vi "AutoDrive.vi"(6 "Distance (Inches)":dbl, 7 "GyroDevRef":T6={"DevStatus"={"status"=FALSE, "code"=0, "source"=""}, "Analog Channel"=enum."AI 0", "Gain (VoltsPerDegree/Second)"=0.0, "Gyro Type"=enum."Analog", "Handle"=0, "SPI Bus"=enum."Invalid", "Device Found"=FALSE, "Sample Rate"=1.0, "Calibrate On Open"=FALSE, "Offset"=0.0} {"Sample Rate" min=0.25 max=100.0 step=0.25}, 8 "error in":errorcluster, 9 "LeftDevRef":T1={"DeviceStatus"={"status"=FALSE, "code"=0, "source"=""}, "Type"=enum."PWM", "PWM"={"PWM Channel"=enum."PWM 1", "DeadBand"={"Name"="", "maxPositivePwm"=0, "minPositivePwm"=0, "centerPwm"=0, "maxNegativePwm"=0, "minNegativePwm"=0, "angularRange"=0}}, "CAN"={"Device Number"=0, "SetOutput VI Ref"=variant(enum8{"Percent VBus", "Current", "Speed", "Position", "Voltage"} enum."Percent VBus"), "GetOutput VI Ref"=variant(refnum<k1> refnum), "Enable VI Ref"=variant(dbl 12.0), "Disable VI Ref"=variant(enum8{"Percent VBus", "Speed", "Position", "Slave", "Unchanged / Invalid", "Voltage Compensation", "Current", "Motion Profile"} enum."Percent VBus"), "Data"=variant}, "Invert"=FALSE, "DIO PWM"={"PWM \"Enable\" Channel"=enum."Invalid", "DIOChannel"=enum."Invalid", "PWM Rate"=0.0}}, 10 "RightDevRef":T1={"DeviceStatus"={"status"=FALSE, "code"=0, "source"=""}, "Type"=enum."PWM", "PWM"={"PWM Channel"=enum."PWM 1", "DeadBand"={"Name"="", "maxPositivePwm"=0, "minPositivePwm"=0, "centerPwm"=0, "maxNegativePwm"=0, "minNegativePwm"=0, "angularRange"=0}}, "CAN"={"Device Number"=0, "SetOutput VI Ref"=variant(enum8{"Percent VBus", "Current", "Speed", "Position", "Voltage"} enum."Percent VBus"), "GetOutput VI Ref"=variant(refnum<k1> refnum), "Enable VI Ref"=variant(dbl 12.0), "Disable VI Ref"=variant(enum8{"Percent VBus", "Speed", "Position", "Slave", "Unchanged / Invalid", "Voltage Compensation", "Current", "Motion Profile"} enum."Percent VBus"), "Data"=variant}, "Invert"=FALSE, "DIO PWM"={"PWM \"Enable\" Channel"=enum."Invalid", "DIOChannel"=enum."Invalid", "PWM Rate"=0.0}}, 11 "DriveDevRef":T9={"DevStatus"={"status"=FALSE, "code"=0, "source"=""}, "Motors[]"=[], "Square Inputs"=FALSE, "Max Output"=1.0}) -> (0 "error out":errorcluster)   [LabVIEW 2017]
uses:
  <vilib>/Rock Robotics/WPI/RobotDrive/WPI_RobotDriveDevRef.ctl
  <vilib>/Rock Robotics/WPI/MotorControl/WPI_MotorControlDeviceRef.ctl
  <vilib>/Rock Robotics/WPI/MotorControl/WPI_MotorControlType.ctl
  <vilib>/Rock Robotics/SystemInterfaces/DIO/FPGA_DIOPWMChannel.ctl
  <vilib>/Rock Robotics/WPI/PWM/WPI_PWMDeadband.ctl
  <vilib>/Rock Robotics/SystemInterfaces/DIO/FPGA_DIOChannel.ctl
  <vilib>/Rock Robotics/WPI/Gyro/WPI_GyroDevRef.ctl
  <vilib>/Rock Robotics/SystemInterfaces/AI/FPGA_AIChannel.ctl
  <vilib>/Rock Robotics/SystemInterfaces/spilib/spi_bus.ctl
  <vilib>/Rock Robotics/WPI/ThirdParty/Phoenix-LabVIEW/Motor Controller/Get/CTRE_Phoenix_MotorController_GetQuadratureData.vi
  <vilib>/Rock Robotics/WPI/RobotDrive/WPI_RobotDriveArcadeDrive_Standard(NoSaturation).vi
panel:
  # "Analog"
  # "XRS"
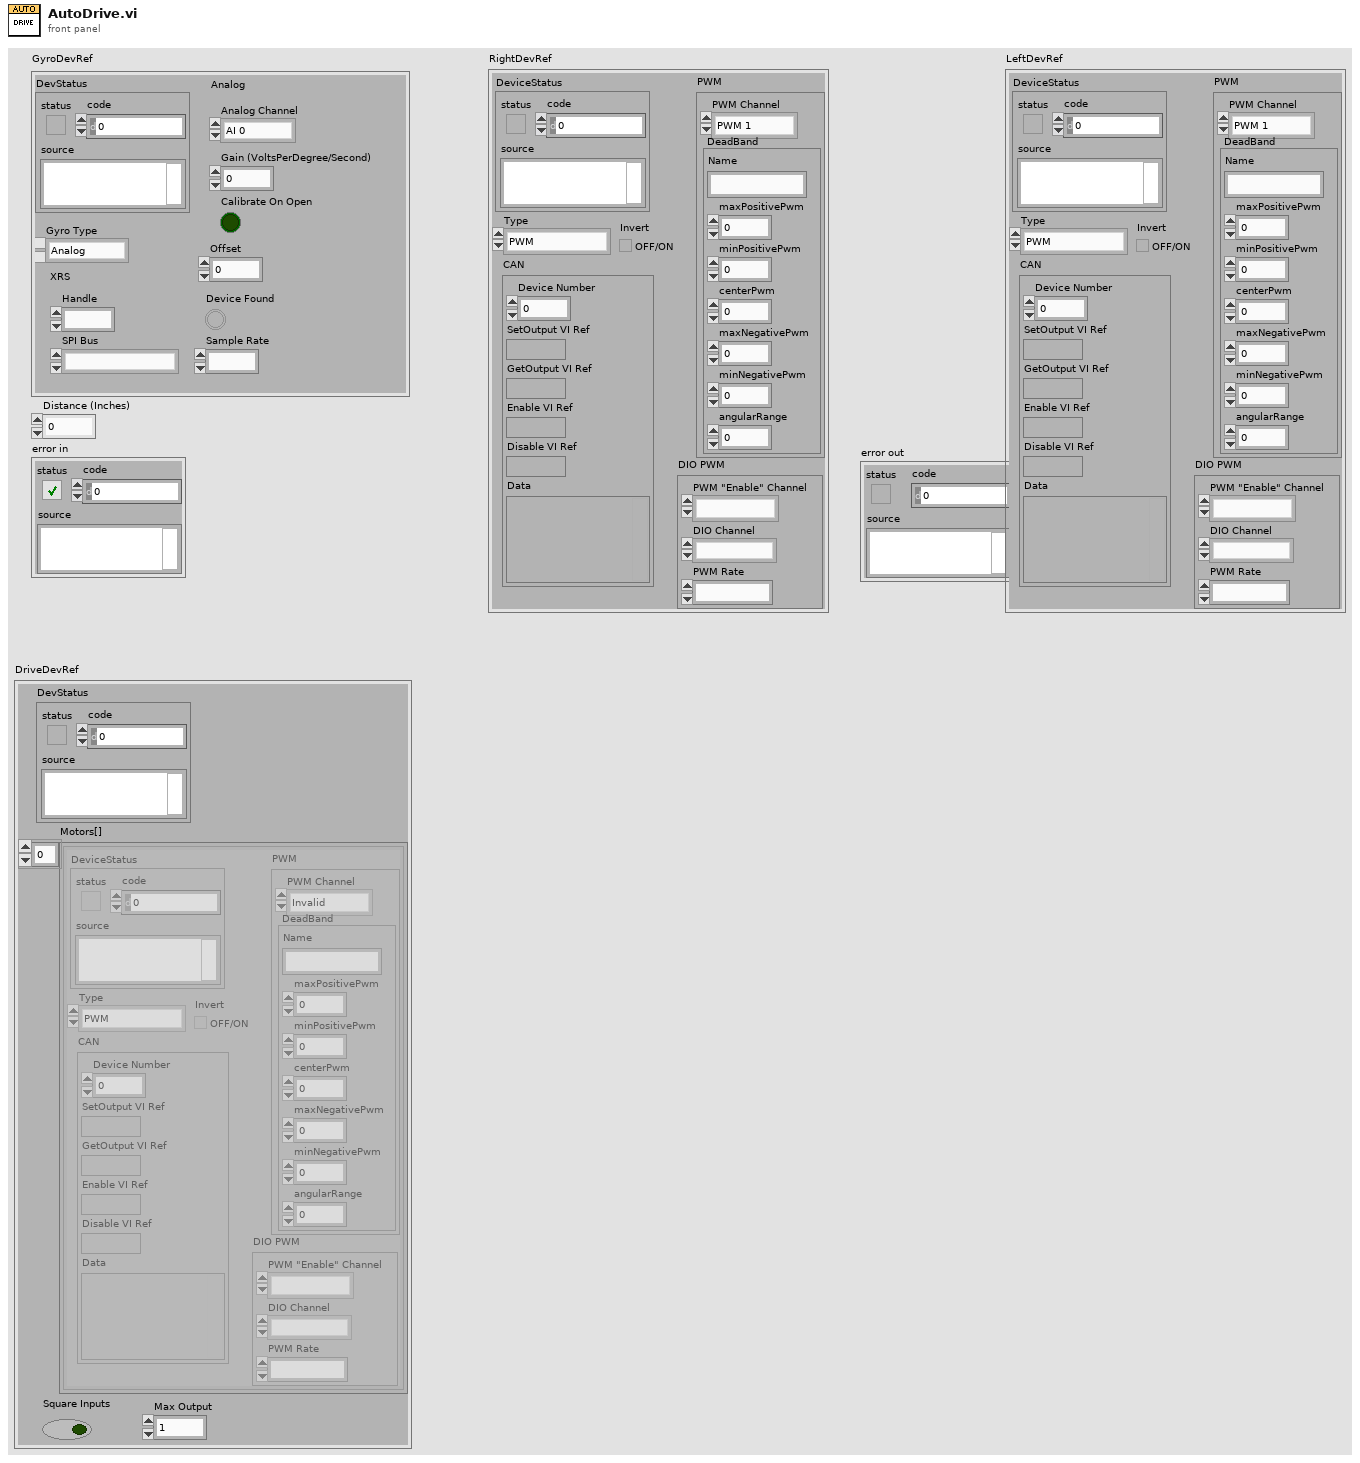
[diagram p1: front panel]
types:
  T1 = typedef "WPI_MotorControlDeviceRef.ctl" = cluster{"DeviceStatus":errorcluster, "Type":T2, "PWM":cluster{"PWM Channel":T3, "DeadBand":T4}, "CAN":cluster{"Device Number":u8, "SetOutput VI Ref":variant, "GetOutput VI Ref":variant, "Enable VI Ref":variant, "Disable VI Ref":variant, "Data":variant}, "Invert":bool, "DIO PWM":cluster{"PWM \"Enable\" Channel":T3, "DIOChannel":T5, "PWM Rate":dbl}}
  T2 = typedef "WPI_MotorControlType.ctl" = enum16{"PWM", "CAN", "DIO PWM"}
  T3 = typedef "FPGA_DIOPWMChannel.ctl" = enum8{"PWM 0", "PWM 1", "PWM 2", "PWM 3", "PWM 4", "PWM 5", "PWM 6", "PWM 7", "PWM 8", "PWM 9", "PWM MXP 0", "PWM MXP 1", "PWM MXP 2", "PWM MXP 3", "PWM MXP 4", "PWM MXP 5", "PWM MXP 6", "PWM MXP 7", "PWM MXP 8", "PWM MXP 9", "Invalid"}
  T4 = typedef "WPI_PWMDeadband.ctl" = cluster{"Name":string, "maxPositivePwm":i32, "minPositivePwm":i32, "centerPwm":i32, "maxNegativePwm":i32, "minNegativePwm":i32, "angularRange":u16}
  T5 = typedef "FPGA_DIOChannel.ctl" = enum8{"DIO 0", "DIO 1", "DIO 2", "DIO 3", "DIO 4", "DIO 5", "DIO 6", "DIO 7", "DIO 8", "DIO 9", "DIO MXP 0", "DIO MXP 1", "DIO MXP 2", "DIO MXP 3", "DIO MXP 4", "DIO MXP 5", "DIO MXP 6", "DIO MXP 7", "DIO MXP 8", "DIO MXP 9", "DIO MXP 10", "DIO MXP 11", "DIO MXP 12", "DIO MXP 13", "DIO MXP 14", "DIO MXP 15", "SPI Port CS1", "SPI Port CS2", "SPI Port CS3", "SPI Port MISO", "SPI Port MOSI", "Invalid"}
  T6 = typedef "WPI_GyroDevRef.ctl" = cluster{"DevStatus":errorcluster, "Analog Channel":T7, "Gain (VoltsPerDegree/Second)":dbl, "Gyro Type":enum16{"Analog", "XRS450"}, "Handle":i32, "SPI Bus":T8, "Device Found":bool, "Sample Rate":dbl, "Calibrate On Open":bool, "Offset":dbl}
  T7 = typedef "FPGA_AIChannel.ctl" = enum8{"AI 0", "AI 1", "AI 2", "AI 3", "AI MXP 0", "AI MXP 1", "AI MXP 2", "AI MXP 3", "Invalid"}
  T8 = typedef "spi_bus.ctl" = enum16{"SPI On-Board, CS0", "SPI On-Board, CS1", "SPI On-Board, CS2", "SPI On-Board, CS3", "SPI MXP", "Invalid"}
  T9 = typedef "WPI_RobotDriveDevRef.ctl" = cluster{"DevStatus":errorcluster, "Motors[]":T1[], "Square Inputs":bool, "Max Output":dbl}
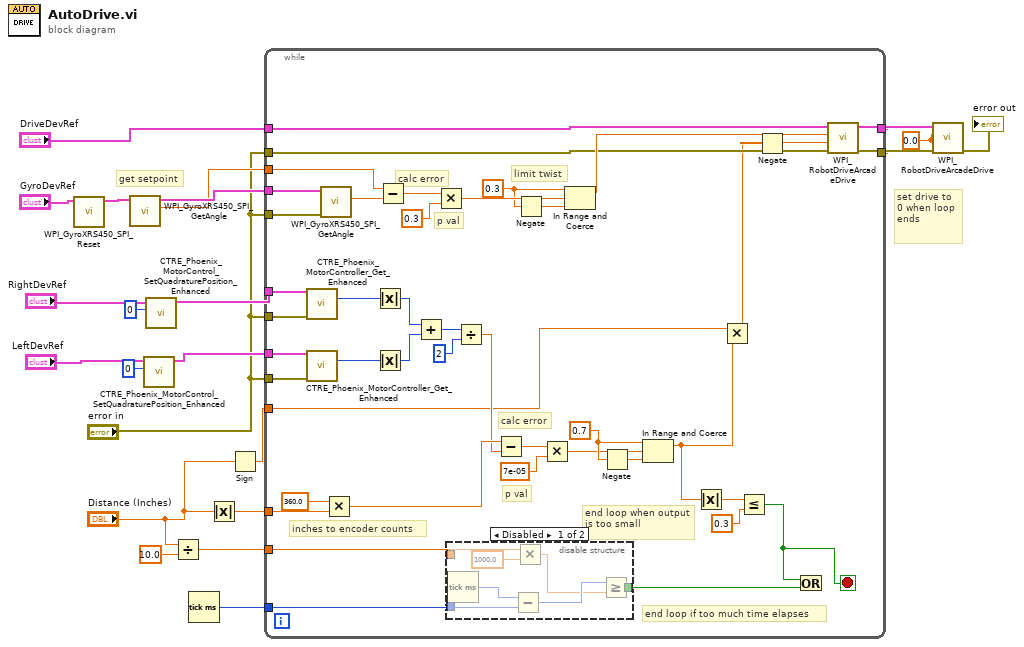
[diagram p0: block diagram]
diagram:
  w13 = 0.0 ("Y axis value")
  # "set drive to 0 when loop ends"
  # "get setpoint"
  n1 = call <vilib>:"WPI_GyroXRS450_SPI_Reset.vi"("GyroDevRef"="GyroDevRef") -> ("GyroDevRef"=w6:T6)  [unwired: 9 in, 1 out]
  n2 = call <vilib>:"WPI_GyroXRS450_SPI_GetAngle.vi"("GyroDevRef"=w6) -> ("Angle"=w16:dbl, "GyroDevRef"=w17:T6)  [unwired: 6 in, 3 out]
  n3 = call <vilib>:"CTRE_Phoenix_MotorControl_SetQuadraturePosition_Enhanced.vi"("New Position"=0, "PhoenixMotorControlDevRef"="LeftDevRef") -> ("PhoenixMotorControlDevRef"=w20:T1)  [unwired: 8 in, 1 out]
  n4 = call <vilib>:"CTRE_Phoenix_MotorControl_SetQuadraturePosition_Enhanced.vi"("New Position"=0, "PhoenixMotorControlDevRef"="RightDevRef") -> ("PhoenixMotorControlDevRef"=w21:T1)  [unwired: 8 in, 1 out]
  n5 = Divide(x="Distance (Inches)", y=10.0) -> (x/y=w1:dbl)
  n6 = Tick Count (ms)() -> (millisecond timer value=w2:u32)
  n7 = Absolute Value(x="Distance (Inches)") -> (abs(x)=w8:dbl)
  n8 = Sign(1:"Distance (Inches)") -> (0:w7:dbl)
  n9 = while {
    tunnel: w8 -> [w65]
    tunnel: w21 -> [w64]
    tunnel: w20 -> [w63]
    tunnel: w17 -> [w55]
    tunnel: "error in" -> [w54]
    tunnel: "error in" -> [w53]
    tunnel: "error in" -> [w52]
    tunnel: "error in" -> [w51]
    tunnel: "DriveDevRef" -> [w50]
    tunnel: w16 -> [w44]
    tunnel: [w36] -> w15
    tunnel: [w35] -> w14
    tunnel: w7 -> [w27]
    tunnel: w2 -> [w26]
    tunnel: w1 -> [w25]
    stop <- w23 stop-if-true
    w30 = 0.7 ("upper limit")
    w32 = 0.3 ("upper limit")
    # "end loop if too much time elapses"
    # "p val"
    # "calc error"
    # "end loop when output is too small"
    # "inches to encoder counts"
    # "limit twist"
    # "p val"
    # "calc error"
    n10 = call-poly <vilib>:"CTRE_Phoenix_MotorController_Get_Enhanced.vi"("PhoenixMotorControlDevRef"=w64, "error in"=w54) -> ("Quadrature Position"=w49:i32)  [unwired: 10 in, 3 out]
    n11 = call-poly <vilib>:"CTRE_Phoenix_MotorController_Get_Enhanced.vi"("PhoenixMotorControlDevRef"=w63, "error in"=w51) -> ("Quadrature Position"=w48:i32)  [unwired: 10 in, 3 out]
    n12 = call <vilib>:"WPI_GyroXRS450_SPI_GetAngle.vi"("error in"=w53, "GyroDevRef"=w55) -> ("Angle"=w47:dbl)  [unwired: 5 in, 4 out]
    n13 = Multiply(x=360.0 ("convert"), y=w65) -> (x*y=w42:dbl)
    n14 = Absolute Value(x=w49) -> (abs(x)=w62:i32)
    n15 = Absolute Value(x=w48) -> (abs(x)=w61:i32)
    n16 = Subtract(x=w44, y=w47) -> (x-y=w58:dbl)
    n17 = Add(x=w62, y=w61) -> (x+y=w60:i32)
    n18 = Multiply(x=w58, y=0.3 ("x")) -> (x*y=w46:dbl)
    n19 = disable-structure shown="Disabled" {
      disable-tunnel: w26 -> [w71 _]
      disable-tunnel: w25 -> [w70 _]
      disable-tunnel: [w66 _] -> w24
      frame Disabled {
        n20 = Tick Count (ms)() -> (millisecond timer value=w72:u32)
        n21 = Subtract(x=w72, y=w71) -> (x-y=w68:u32)
        n22 = Multiply(x=w70, y=1000.0) -> (x*y=w67:dbl)
        n23 = Greater Or Equal?(x=w68, y=w67) -> (x >= y?=w66:bool)
      }
      frame Enabled {
      }
    }
    n24 = Divide(x=w60, y=2) -> (x/y=w41:dbl)
    n25 = Subtract(x=w42, y=w41) -> (x-y=w38:dbl)
    n26 = Negate(x=w32) -> (-x=w33:dbl)
    n27 = Multiply(x=w38, y=7e-05) -> (x*y=w29:dbl)
    n28 = In Range and Coerce(upper limit=w32, x=w46, lower limit=w33) -> (coerced(x)=w56:dbl)  [unwired: 1 out]
    n29 = Negate(x=w30) -> (-x=w31:dbl)
    n30 = In Range and Coerce(upper limit=w30, x=w29, lower limit=w31) -> (coerced(x)=w34:dbl)  [unwired: 1 out]
    n31 = Absolute Value(x=w34) -> (abs(x)=w40:dbl)
    n32 = Multiply(x=w27, y=w34) -> (x*y=w28:dbl)
    n33 = Less Or Equal?(x=w40, y=0.3) -> (x <= y?=w23:bool)
    n34 = Negate(x=w28) -> (-x=w37:dbl)
    n35 = Or(x=w23, y=w24) -> ()  [unwired: 1 out]
    n36 = call-poly <vilib>:"WPI_RobotDriveArcadeDrive.vi"("error in (no error)"=w52, "Y axis value"=w37, "X axis value"=w56, "RobotDriveDevRef"=w50) -> ("error out"=w35:errorcluster, "RobotDriveDevRef"=w36:T9)  [unwired: 5 in, 1 out]
  }
  n37 = call-poly <vilib>:"WPI_RobotDriveArcadeDrive.vi"("error in (no error)"=w14, "Y axis value"=w13, "X axis value"=w13, "RobotDriveDevRef"=w15) -> ("error out"=→"error out":errorcluster)  [unwired: 5 in, 2 out]
